vi "ControlGraphMove.vi"(10 "x":dbl, 11 "ref xy graph":refnum<vi>) -> ()   [LabVIEW 2018]
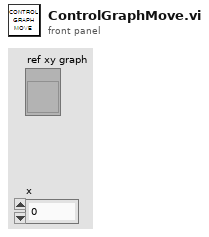
[diagram p1: front panel]
types:
  T1 = typedef "LVPoint32TypeDef.ctl" = cluster{"Horizontal":i32, "Vertical":i32}
  T2 = typedef "LVRectTypeDef.ctl" = cluster{"Left":i16, "Top":i16, "Right":i16, "Bottom":i16}
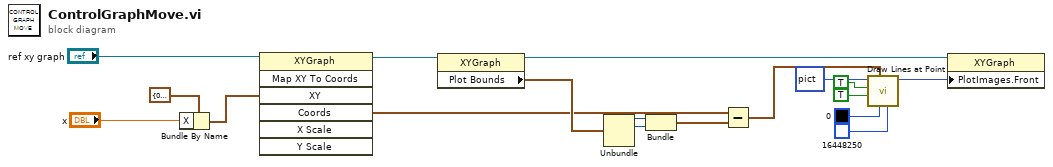
[diagram p0: block diagram]
diagram:
  n1 = Bundle By Name(cluster=cluster{"X":dbl, "Y":dbl} {"X"=0.0, "Y"=0.0} ("XY"), "X"="x") -> (w10:cluster{"X":dbl, "Y":dbl})
  n2 = invoke on="Invoke Node" class="XYGraph" method="Map XY To Coords"(reference="ref xy graph", "XY"=w10) -> (reference out=w15:refnum<vi>, "Coords"=w13:T1)  [unwired: 5 in, 5 out]
  n3 = property class="XYGraph"(reference=w15) -> (reference out=w12:refnum<vi>, "Plot Bounds"=w14:T2)  [unwired: 1 in, 1 out]
  n4 = Unbundle(w14) -> ("Left"=w17:i16, "Top"=w18:i16)  [unwired: 2 out]
  n5 = Bundle("Left"=w17, "Top"=w18) -> (w16:cluster{"Left":i16, "Top":i16})  [unwired: 1 in]
  n6 = Subtract(x=w13, y=w16) -> (x-y=w8:T1)
  n7 = call "Draw Lines at Point.vi"("GraphBGK"=u32 16448250, "color(black)"=u32 0, "pixel center"=w8, "Vertical Line?"=TRUE, "Horizontal Line?"=TRUE, "new picture in"=picture data[5B]) -> ("new picture out"=w7:picture)  [unwired: 5 in]
  n8 = property class="XYGraph"(reference=w12, "PlotImages.Front"=w7) -> ()  [unwired: 1 in, 2 out]
